vi "Get LRS Data.vi"(8 "error in":errorcluster, 11 "tCRD in":refnum<class "Aircraft OPCCRD.lvclass">) -> (0 "error out":errorcluster, 3 "tCRD out":refnum<class "Aircraft OPCCRD.lvclass">)   [LabVIEW 2015, in "Aircraft OPCCRD.lvclass"]
uses:
  Aircraft OPCCRD.lvclass
  Aircraft OPCCRD.lvclass/Aircraft OPCCRD.ctl
  Reusable/CRDS/Main/CRDS.lvclass/CRDS.ctl
  Reusable/CRDS/Cell/CRDS Cell.lvclass/CRDS Cell.ctl
  Reusable/CRDS/Data/Cell/CRDS Cell Data.lvclass/CRDS Cell Data.ctl
  Accessors/Read FPGA Ref.vi
  Accessors/Read RepRate.vi
  Reusable/CRDS/Main/Read writeRDs.vi
  Reusable/CRDS/Cell/Read NumTaus.vi
  Reusable/CRDS/Cell/Read Data.vi
  Reusable/CRDS/Data/Cell/Read extParam.vi
  Reusable/CRDS/Main/Read Cells.vi
  Reusable/CRDS/Cell/Read dt.vi
  <vilib>/Utility/error.llb/Error Cluster From Error Code.vi
  <vilib>/rvi/errors/niLvFpgaAdjustHostInterfaceError.vi
  tFPGA Ref.ctl
  Reusable/CRDS/Cell/CRDS Cell.lvclass
  Reusable/CRDS/Data/Cell/CRDS Cell Data.lvclass
  <vilib>/rvi/interface/nirviReadWriteControl/nirviReadWriteControl.xnode
  FPGA Bitfiles/Aircraft OPCRD Server.lvbitx
  <vilib>/rvi/interface/nirviMethod/nirviMethod.xnode
  NiFpgaLv.dll
  <vilib>/FPGAPlugInAG/sbRIO-9636/niLvFpga_ReadFifo_sbRIO-9636.vi
  <vilib>/rvi/errors/niLvFpgaMergeErrorWithErrorCode.vi
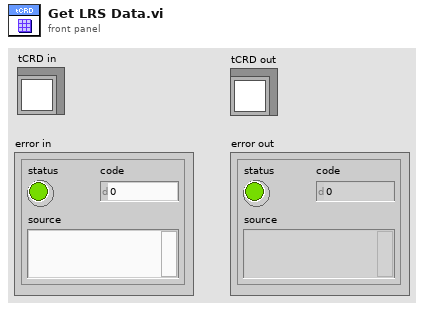
[diagram p1: front panel]
types:
  T1 = typedef "Aircraft OPCCRD.lvclass/tFPGA Ref.ctl" = refnum<k20>
  T2 = typedef "extparam.ctl" = cluster{"Tau":sgl, "Tau0cor":sgl, "ext":sgl, "extCorr":sgl, "stdevTau":sgl, "eTau":sgl, "taucorr":sgl, "Tau0":sgl, "max":sgl}
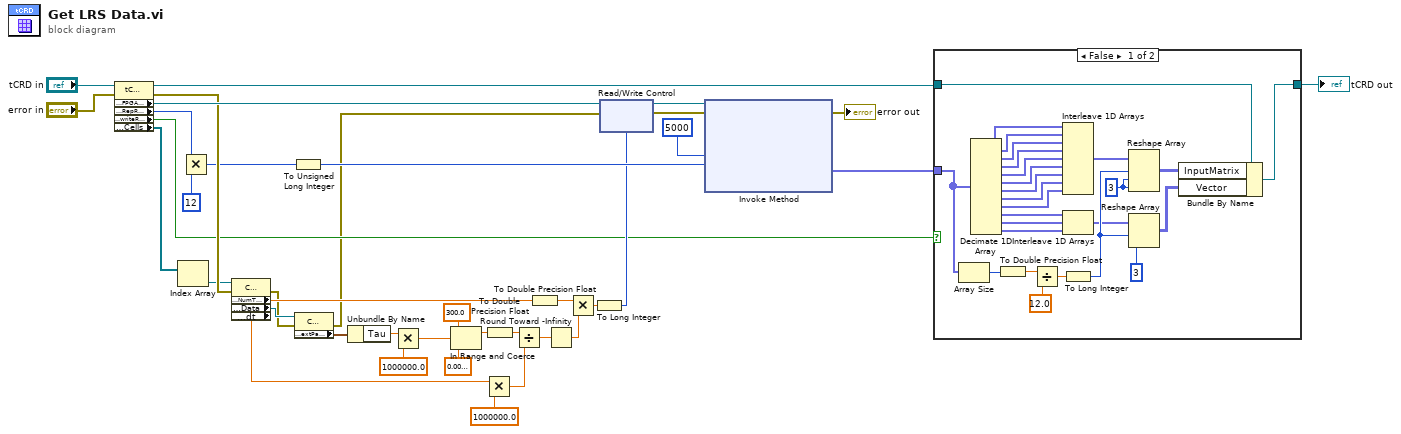
[diagram p0: block diagram]
diagram:
  n1 = property class="tCRD"(reference="tCRD in", error in="error in") -> (reference out=w37:refnum<class "Aircraft OPCCRD.lvclass">, error out=w34:errorcluster, "Accessors:FPGA Ref"=w36:T1, "Accessors:RepRate"=w35:u16, "Accessors:writeRDs"=w6:bool, "Data Access:Cells"=w5:refnum<class "CRDS Cell.lvclass">[])
  n2 = Index Array(array=w5) -> (element=w18:refnum<class "CRDS Cell.lvclass">)  [unwired: 1 in]
  n3 = Multiply(x=w35, y=u16 12) -> (x*y=w28:u16)
  n4 = property class="CRDS Cell"(reference=w18, error in=w34) -> (error out=w4:errorcluster, "Data Access:NumTaus"=w30:sgl, "Data Access:Data"=w19:refnum<class "CRDS Cell Data.lvclass">, "Data Access:dt"=w3:dbl)  [unwired: 1 out]
  n5 = To Unsigned Long Integer(number=w28) -> (unsigned 32bit integer=w29:u32)
  n6 = property class="CRDS Cell"(reference=w19, error in=w4) -> (error out=w2:errorcluster, "Data Access:extParam"=w20:T2)  [unwired: 1 out]
  n7 = Unbundle By Name(w20) -> ("Tau"=w32:sgl)
  n8 = Multiply(x=w32, y=sgl 1000000.0) -> (x*y=w11:sgl)
  n9 = In Range and Coerce(upper limit=sgl 300.0, x=w11, lower limit=sgl 0.01) -> (coerced(x)=w8:sgl)  [unwired: 1 out]
  n10 = Multiply(x=w3, y=1000000.0) -> (x*y=w22:dbl)
  n11 = To Double Precision Float(number=w8) -> (double precision float=w7:dbl)
  n12 = Divide(x=w7, y=w22) -> (x/y=w17:dbl)
  n13 = To Double Precision Float(number=w30) -> (double precision float=w27:dbl)
  n14 = Round Toward -Infinity(1:w17) -> (0:w16:dbl)
  n15 = Multiply(x=w27, y=w16) -> (x*y=w15:dbl)
  n16 = To Long Integer(number=w15) -> (32bit integer=w24:i32)
  n17 = xnode "Read/Write Control"("FPGA VI Reference In"=w36, "error in"=w2, "max"=w24) -> ("FPGA VI Reference Out"=w23:T1, "error out"=w26:errorcluster)
  n18 = xnode "Invoke Method"("FPGA VI Reference In"=w23, "error in"=w26, "Number of Elements"=w29, "Timeout (ms)"=5000) -> ("error out"=→"error out":errorcluster, "Data"=w25:fxp<+/-,64,64>[])  [unwired: 2 out]
  n19 = case shown="False" w6 {
    tunnel: [w64 w65] -> w1
    tunnel: w37 -> [w63 w65]
    tunnel: w25 -> [w62 _]
    frame False {
      w58 = 3 ("dimension size")
      n20 = Array Size(array=w62) -> (size(s)=w59:i32)
      n21 = Decimate 1D Array(w62) -> (w41:fxp<+/-,64,64>[], w42:fxp<+/-,64,64>[], w43:fxp<+/-,64,64>[], w44:fxp<+/-,64,64>[], w45:fxp<+/-,64,64>[], w46:fxp<+/-,64,64>[], w47:fxp<+/-,64,64>[], w48:fxp<+/-,64,64>[], w49:fxp<+/-,64,64>[], w52:fxp<+/-,64,64>[], w50:fxp<+/-,64,64>[], w51:fxp<+/-,64,64>[])
      n22 = To Double Precision Float(number=w59) -> (double precision float=w60:dbl)
      n23 = Divide(x=w60, y=12.0) -> (x/y=w55:dbl)
      n24 = Interleave 1D Arrays(w41, w42, w43, w44, w45, w46, w47, w48, w49) -> (w56:fxp<+/-,64,64>[])
      n25 = Interleave 1D Arrays(w52, w50, w51) -> (w53:fxp<+/-,64,64>[])
      n26 = To Long Integer(number=w55) -> (32bit integer=w57:i32)
      n27 = Reshape Array(w56, w57, w58, w58) -> (w40:fxp<+/-,64,64>[][][])
      n28 = Reshape Array(w53, w57, 3 ("dimension size")) -> (w39:fxp<+/-,64,64>[][])
      n29 = Bundle By Name(cluster=w63, "InputMatrix"=w40, "Vector"=w39) -> (w64:refnum<class "Aircraft OPCCRD.lvclass">)
    }
    frame True {
    }
  }
  "tCRD out" <- w1
